vi "read value.vi"(8 "error in (no error)":errorcluster, 11 "File interpreter in":refnum<class "File interpreter.lvclass">) -> (0 "error out":errorcluster, 2 "value":string, 3 "File interpreter out":refnum<class "File interpreter.lvclass">)   [LabVIEW 2018, in "File interpreter.lvclass"]
uses:
  File interpreter.lvclass
  File interpreter.lvclass/File interpreter.ctl
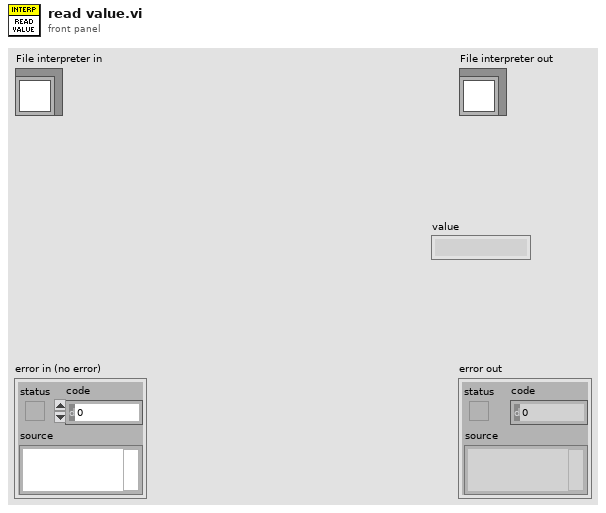
[diagram p1: front panel]
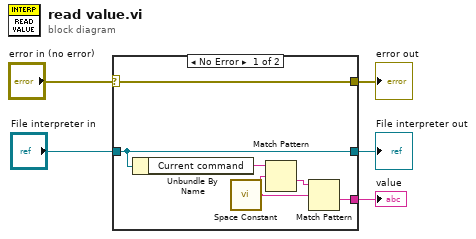
[diagram p0: block diagram]
diagram:
  n1 = case shown="No Error" "error in (no error)" {
    selector: "error in (no error)" -> [w11 w13]
    tunnel: [w11 w13] -> w4
    tunnel: [w10 w12] -> w2
    tunnel: "File interpreter in" -> [w10 w12]
    tunnel: [w6 _] -> w1
    frame No Error {
      n2 = Unbundle By Name(w10) -> ("Current command"=w9:string)
      n3 = call <vilib>:"Space Constant.vi"() -> ("String"=w7:string)
      n4 = Match Pattern(string=w9, regular expression=w7) -> (after substring=w8:string)  [unwired: 1 in, 3 out]
      n5 = Match Pattern(string=w8, regular expression=w7) -> (after substring=w6:string)  [unwired: 1 in, 3 out]
    }
    frame Error {
    }
  }
  "error out" <- w4
  "File interpreter out" <- w2
  "value" <- w1
